vi "Initialize Attributes Core.vi"(8 "error in (no error)":errorcluster, 10 "Attribute Data":variant, 11 "BNT_ULx-MCSV-DOPWM in":refnum<class "BNT_ULx-MCSV-DOPWM.lvclass">) -> (0 "error out":errorcluster, 2 "MandatoryParameters":cluster{"Parameter":string, "found?":bool}[](array[cluster]), 3 "BNT_ULx-MCSV-DOPWM out":refnum<class "BNT_ULx-MCSV-DOPWM.lvclass">)   [LabVIEW 2020, in "BNT_ULx.lvlib" / "BNT_ULx-MCSV-DOPWM.lvclass"]
doc: "Initialize object attribute.\n\nUnique resources should be allocated elsewhere!"
uses:
  BNT_ULx-MCSV-DOPWM.lvclass
  C:/User/Brand/LVP/CSPP/CSPP-Template/Packages/CSPP_Core/Actors/CSPP_BaseActor/CSPP_BaseActor.lvclass
  CSPP_Core/Actors/CSPP_BaseActor/CSPP_BaseActor.lvclass/CSPP_BaseActor.ctl
  BNT_ULx-MCSV-DOPWM.lvclass/BNT_ULx-MCSV-DOPWM.ctl
  BNT_ULx-MCSV/BNT_ULx-MCSV.lvclass
  CSPP_Core/Classes/CSPP_BaseClasses/Factory/CSPP_Factory.lvclass
  CSPP_Core/Actors/CSPP_BaseActor/CSPP_BaseActor.lvclass
  CSPP_Core/Classes/CSPP_ProcessVariables/CSPP_ProcessVariables.lvlib
  CSPP_Core/Libraries/Utilities/CSPP_Utilities.lvlib
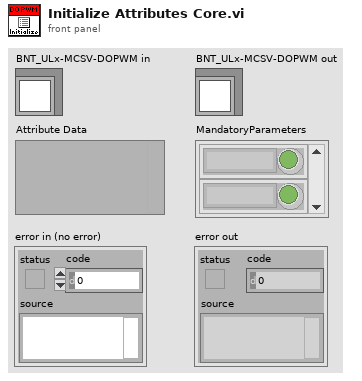
[diagram p1: front panel]
types:
  T1 = cluster{string, "Type Descriptor":string, string}
  T2 = cluster{"initial string":string, "Type Descriptor":string, string}
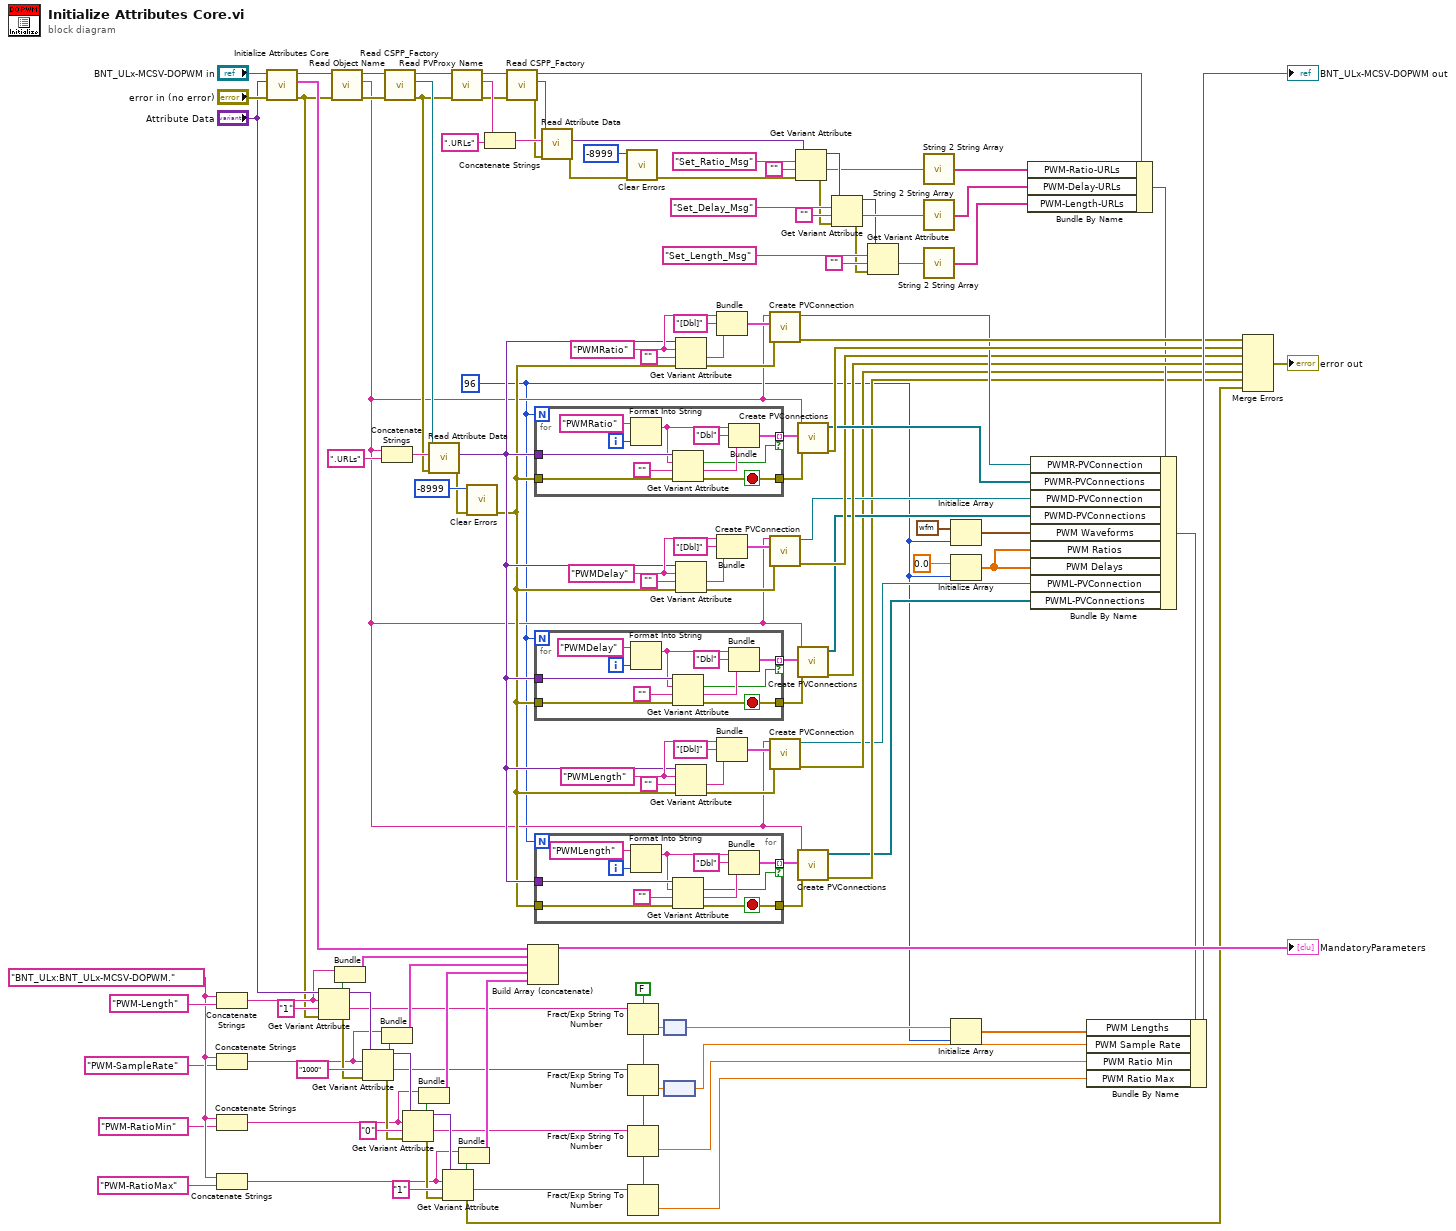
[diagram p0: block diagram]
diagram:
  w18 = "PWMLength" ("initial string")
  w59 = "PWMDelay" ("initial string")
  w73 = "PWMRatio" ("initial string")
  w7 = 96
  w77 = FALSE ("use system decimal point (T)")
  w119 = "BNT_ULx:BNT_ULx-MCSV-DOPWM."
  n1 = Concatenate Strings(w119, "PWM-Length" ("string")) -> (w126:string)
  n2 = Concatenate Strings(w119, "PWM-SampleRate" ("string")) -> (w108:string)
  n3 = Concatenate Strings(w119, "PWM-RatioMin" ("string")) -> (w107:string)
  n4 = Concatenate Strings(w119, "PWM-RatioMax" ("string")) -> (w105:string)
  n5 = call-parent "Initialize Attributes Core.vi"("error in (no error)"="error in (no error)", "Attribute Data"="Attribute Data", "BNT_ULx-MCSV in"="BNT_ULx-MCSV-DOPWM in") -> ("error out"=w82:errorcluster, "MandatoryParameters"=w132:cluster{"Parameter":string, "found?":bool}[], "BNT_ULx-MCSV out"=w83:refnum<class "BNT_ULx-MCSV-DOPWM.lvclass">)  [unwired: 6 in]
  n6 = Get Variant Attribute(Variant="Attribute Data", name=w126, default value (empty Variant)="1" ("string"), error in=w82) -> (duplicate Variant=w115:variant, found=w125:bool, value=w100:string, error out=w114:errorcluster)
  n7 = call "Read Object Name.vi"("error in (no error)"=w82, "CSPP_BaseActor in"=w83) -> ("error out"=w84:errorcluster, "Object Name"=w12:string, "CSPP_BaseActor out"=w90:refnum<class "BNT_ULx-MCSV-DOPWM.lvclass">)  [unwired: 7 in]
  n8 = Bundle(w126, w125) -> (w124:cluster{string, bool})  [unwired: 1 in]
  n9 = Get Variant Attribute(Variant=w115, name=w108, default value (empty Variant)="1000" ("string"), error in=w114) -> (duplicate Variant=w113:variant, found=w109:bool, value=w96:string, error out=w112:errorcluster)
  n10 = Concatenate Strings(w12, ".URLs" ("string")) -> (w88:string)
  n11 = Bundle(w108, w109) -> (w103:cluster{string, bool})  [unwired: 1 in]
  n12 = call "Read CSPP_Factory.vi"("error in (no error)"=w84, "CSPP_BaseActor in"=w90) -> ("error out"=w30:errorcluster, "CSPP_Factory"=w85:refnum<class "CSPP_Factory.lvclass">, "CSPP_BaseActor out"=w31:refnum<class "BNT_ULx-MCSV-DOPWM.lvclass">)  [unwired: 7 in]
  n13 = Get Variant Attribute(Variant=w113, name=w107, default value (empty Variant)="0" ("string"), error in=w112) -> (duplicate Variant=w111:variant, found=w106:bool, value=w95:string, error out=w110:errorcluster)
  n14 = Bundle(w107, w106) -> (w102:cluster{string, bool})  [unwired: 1 in]
  n15 = call-dynamic "Read Attribute Data.vi"("error in (no error)"=w30, "Object Name"=w88, "CSPP_Factory in"=w85) -> ("error out"=w86:errorcluster, "Attribute Data"=w14:variant)  [unwired: 6 in, 1 out]
  n16 = Get Variant Attribute(Variant=w111, name=w105, default value (empty Variant)="1" ("string"), error in=w110) -> (found=w104:bool, value=w94:string, error out=w78:errorcluster)  [unwired: 1 out]
  n17 = call "Read PVProxy Name.vi"("error in (no error)"=w30, "CSPP_BaseActor in"=w31) -> ("error out"=w32:errorcluster, "PVProxy Name"=w45:string, "CSPP_BaseActor out"=w34:refnum<class "BNT_ULx-MCSV-DOPWM.lvclass">)  [unwired: 7 in]
  n18 = Bundle(w105, w104) -> (w101:cluster{string, bool})  [unwired: 1 in]
  n19 = call <vilib>:"Clear Errors.vi"("error in (no error)"=w86, "specific error code to clear (0: all)"=-8999) -> ("error out"=w13:errorcluster)  [unwired: 4 in, 1 out]
  n20 = Concatenate Strings(w45, ".URLs" ("string")) -> (w47:string)
  n21 = call "Read CSPP_Factory.vi"("error in (no error)"=w32, "CSPP_BaseActor in"=w34) -> ("error out"=w29:errorcluster, "CSPP_Factory"=w33:refnum<class "CSPP_Factory.lvclass">, "CSPP_BaseActor out"=w28:refnum<class "BNT_ULx-MCSV-DOPWM.lvclass">)  [unwired: 7 in]
  n22 = Build Array (concatenate)(w132, w124, w103, w102, w101) -> (→"MandatoryParameters":cluster{"Parameter":string, "found?":bool}[])
  n23 = for {
    N: w7 -> [_]
    tunnel: w14 -> [w142]
    tunnel: w13 -> [w141]
    tunnel: [w137] -> w81 mode=indexing if=w134
    tunnel: [w133] -> w80
    i -> [w140]
    stop <- w133 stop-if-true
    n24 = Format Into String(initial string="PWMRatio", w140) -> (resulting string=w138:string)  [unwired: 2 in, 1 out]
    n25 = Get Variant Attribute(Variant=w142, name=w138, default value (empty Variant)="", error in=w141) -> (found=w134:bool, value=w135:string, error out=w133:errorcluster)  [unwired: 1 out]
    n26 = Bundle(w138, "Type Descriptor"="Dbl", w135) -> (w137:T1)  [unwired: 1 in]
  }
  n27 = for {
    N: w7 -> [_]
    tunnel: w14 -> [w153]
    tunnel: w13 -> [w152]
    tunnel: [w148] -> w55 mode=indexing if=w145
    tunnel: [w144] -> w56
    i -> [w151]
    stop <- w144 stop-if-true
    n28 = Format Into String(initial string="PWMDelay", w151) -> (resulting string=w149:string)  [unwired: 2 in, 1 out]
    n29 = Get Variant Attribute(Variant=w153, name=w149, default value (empty Variant)="", error in=w152) -> (found=w145:bool, value=w146:string, error out=w144:errorcluster)  [unwired: 1 out]
    n30 = Bundle(w149, "Type Descriptor"="Dbl", w146) -> (w148:T1)  [unwired: 1 in]
  }
  n31 = for {
    N: w7 -> [_]
    tunnel: w14 -> [w164]
    tunnel: w13 -> [w163]
    tunnel: [w159] -> w22 mode=indexing if=w156
    tunnel: [w155] -> w21
    i -> [w162]
    stop <- w155 stop-if-true
    n32 = Format Into String(initial string="PWMLength", w162) -> (resulting string=w160:string)  [unwired: 2 in, 1 out]
    n33 = Get Variant Attribute(Variant=w164, name=w160, default value (empty Variant)="", error in=w163) -> (found=w156:bool, value=w157:string, error out=w155:errorcluster)  [unwired: 1 out]
    n34 = Bundle(w160, "Type Descriptor"="Dbl", w157) -> (w159:T1)  [unwired: 1 in]
  }
  n35 = call-dynamic "Read Attribute Data.vi"("error in (no error)"=w29, "Object Name"=w47, "CSPP_Factory in"=w33) -> ("error out"=w49:errorcluster, "Attribute Data"=w43:variant)  [unwired: 6 in, 1 out]
  n36 = call <vilib>:"Clear Errors.vi"("error in (no error)"=w49, "specific error code to clear (0: all)"=-8999) -> ("error out"=w42:errorcluster)  [unwired: 4 in, 1 out]
  n37 = Fract/Exp String To Number(use system decimal point (T)=w77, string=w100) -> (number=w98:dbl)  [unwired: 2 in, 1 out]
  n38 = Fract/Exp String To Number(use system decimal point (T)=w77, string=w96) -> (number=w97:dbl)  [unwired: 2 in, 1 out]
  n39 = Fract/Exp String To Number(use system decimal point (T)=w77, string=w95) -> (number=w92:dbl)  [unwired: 2 in, 1 out]
  n40 = Fract/Exp String To Number(use system decimal point (T)=w77, string=w94) -> (number=w91:dbl)  [unwired: 2 in, 1 out]
  n41 = node(w98) -> (w24:dbl[unit])
  n42 = node(w97) -> (w93:dbl[unit])
  n43 = Get Variant Attribute(Variant=w14, name=w73, default value (empty Variant)="", error in=w13) -> (value=w72:string, error out=w70:errorcluster)  [unwired: 2 out]
  n44 = Get Variant Attribute(Variant=w14, name=w59, default value (empty Variant)="", error in=w13) -> (value=w60:string, error out=w62:errorcluster)  [unwired: 2 out]
  n45 = Get Variant Attribute(Variant=w14, name=w18, default value (empty Variant)="", error in=w13) -> (value=w17:string, error out=w15:errorcluster)  [unwired: 2 out]
  n46 = Bundle("initial string"=w73, "Type Descriptor"="[Dbl]", w72) -> (w71:T2)  [unwired: 1 in]
  n47 = Bundle("initial string"=w59, "Type Descriptor"="[Dbl]", w60) -> (w61:T2)  [unwired: 1 in]
  n48 = Bundle("initial string"=w18, "Type Descriptor"="[Dbl]", w17) -> (w16:T2)  [unwired: 1 in]
  n49 = call "Create PVConnection.vi"("Error In"=w70, "PV-Info"=w71, "Object Name"=w12) -> ("error out"=w69:errorcluster, "PVConnection"=w65:refnum<class "PVConnection.lvclass">)  [unwired: 7 in]
  n50 = call "Create PVConnection.vi"("Error In"=w62, "PV-Info"=w61, "Object Name"=w12) -> ("error out"=w54:errorcluster, "PVConnection"=w52:refnum<class "PVConnection.lvclass">)  [unwired: 7 in]
  n51 = call "Create PVConnection.vi"("Error In"=w15, "PV-Info"=w16, "Object Name"=w12) -> ("error out"=w11:errorcluster, "PVConnection"=w9:refnum<class "PVConnection.lvclass">)  [unwired: 7 in]
  n52 = Get Variant Attribute(Variant=w43, name="Set_Ratio_Msg", default value (empty Variant)="", error in=w42) -> (duplicate Variant=w38:variant, value=w36:string, error out=w37:errorcluster)  [unwired: 1 out]
  n53 = call "Create PVConnections.vi"("Error In"=w80, "PV-Infos"=w81, "Object Name"=w12) -> ("error out"=w79:errorcluster, "PVConnections"=w64:refnum<class "PVConnection.lvclass">[])  [unwired: 7 in]
  n54 = call "Create PVConnections.vi"("Error In"=w56, "PV-Infos"=w55, "Object Name"=w12) -> ("error out"=w53:errorcluster, "PVConnections"=w51:refnum<class "PVConnection.lvclass">[])  [unwired: 7 in]
  n55 = call "Create PVConnections.vi"("Error In"=w21, "PV-Infos"=w22, "Object Name"=w12) -> ("error out"=w10:errorcluster, "PVConnections"=w8:refnum<class "PVConnection.lvclass">[])  [unwired: 7 in]
  n56 = Get Variant Attribute(Variant=w38, name="Set_Delay_Msg", default value (empty Variant)="", error in=w37) -> (duplicate Variant=w3:variant, value=w35:string, error out=w2:errorcluster)  [unwired: 1 out]
  n57 = Get Variant Attribute(Variant=w3, name="Set_Length_Msg", default value (empty Variant)="", error in=w2) -> (value=w6:string)  [unwired: 3 out]
  n58 = call "String 2 String Array.vi"("String"=w36) -> ("Substrings"=w26:string[])  [unwired: 1 in]
  n59 = call "String 2 String Array.vi"("String"=w35) -> ("Substrings"=w25:string[])  [unwired: 1 in]
  n60 = call "String 2 String Array.vi"("String"=w6) -> ("Substrings"=w1:string[])  [unwired: 1 in]
  n61 = Initialize Array(waveform(dbl) {"t0"=timestamp(-9593251200 s since 1904-01-01), "dt"=0.001, "Y"=[]} ("PWM Waveform"), w7) -> (w63:waveform(dbl)[])
  n62 = Initialize Array(0.0 ("PWM Ratio"), w7) -> (w50:dbl[])
  n63 = Initialize Array(w24, w7) -> (w23:dbl[unit][])
  n64 = Bundle By Name(cluster=w28, "PWM-Ratio-URLs"=w26, "PWM-Delay-URLs"=w25, "PWM-Length-URLs"=w1) -> (w27:refnum<class "BNT_ULx-MCSV-DOPWM.lvclass">)
  n65 = Bundle By Name(cluster=w27, "PWMR-PVConnection"=w65, "PWMR-PVConnections"=w64, "PWMD-PVConnection"=w52, "PWMD-PVConnections"=w51, "PWM Waveforms"=w63, "PWM Ratios"=w50, "PWM Delays"=w50, "PWML-PVConnection"=w9, "PWML-PVConnections"=w8) -> (w66:refnum<class "BNT_ULx-MCSV-DOPWM.lvclass">)
  n66 = Bundle By Name(cluster=w66, "PWM Lengths"=w23, "PWM Sample Rate"=w93, "PWM Ratio Min"=w92, "PWM Ratio Max"=w91) -> (→"BNT_ULx-MCSV-DOPWM out":refnum<class "BNT_ULx-MCSV-DOPWM.lvclass">)
  n67 = Merge Errors(w69, w79, w54, w53, w11, w10, w78) -> (→"error out":errorcluster)
